vi "Read 4.vi"(11 "read buffer":string) -> (3 "String":string)   [LabVIEW 2021]
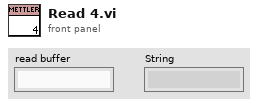
[diagram p1: front panel]
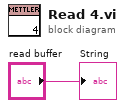
[diagram p0: block diagram]
diagram:
  "String" <- "read buffer"
